vi "Create Cron Expression.vi"(5 "Cron in":refnum<class "Cron.lvclass">, 8 "error in (no error)":errorcluster, 11 "Cron Expression":string) -> (0 "error out":errorcluster, 1 "expression valid":bool, 3 "Cron out":refnum<class "Cron.lvclass">)   [LabVIEW 2013, in "openCron.lvlib" / "Cron.lvclass"]
uses:
  Cron.lvclass
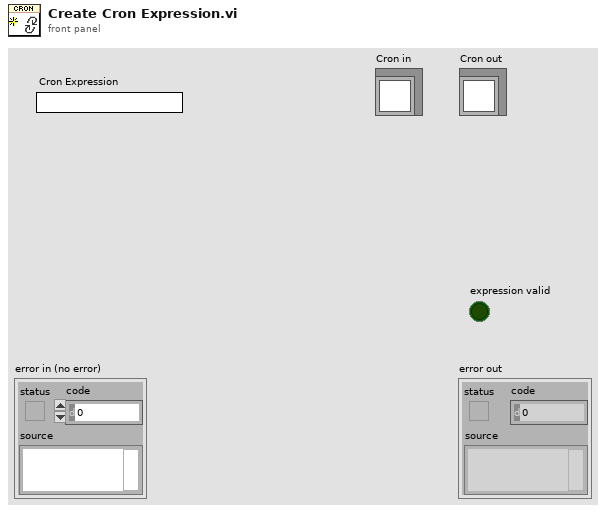
[diagram p1: front panel]
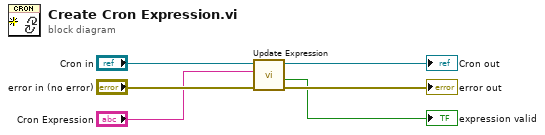
[diagram p0: block diagram]
diagram:
  n1 = call "Update Expression.vi"("error in (no error)"="error in (no error)", "Expression"="Cron Expression", "Cron in"="Cron in") -> ("error out"=→"error out":errorcluster, "valid"=→"expression valid":bool, "Cron out"=→"Cron out":refnum<class "Cron.lvclass">)  [unwired: 6 in]
